vi "Untitled.vi"() -> ()   [LabVIEW 2017, in "Examples.lvlib"]
uses:
  Examples.lvlib
panel:
  in  "Bolts 3":bool
  in  "Bolts 2":bool
  in  "Valve 2":bool
  out "Pipe 2":bool
  in  "OK Button 2":bool
  out "Tank 2":dbl(slide) scale=0.0..10.0
  in  "Stop Button":bool
  out "Pipe":bool
  in  "Tank":bool
  in  "Bolts":bool
  out "Valve":bool
  in  "Switch":bool
  out "Boiler":bool
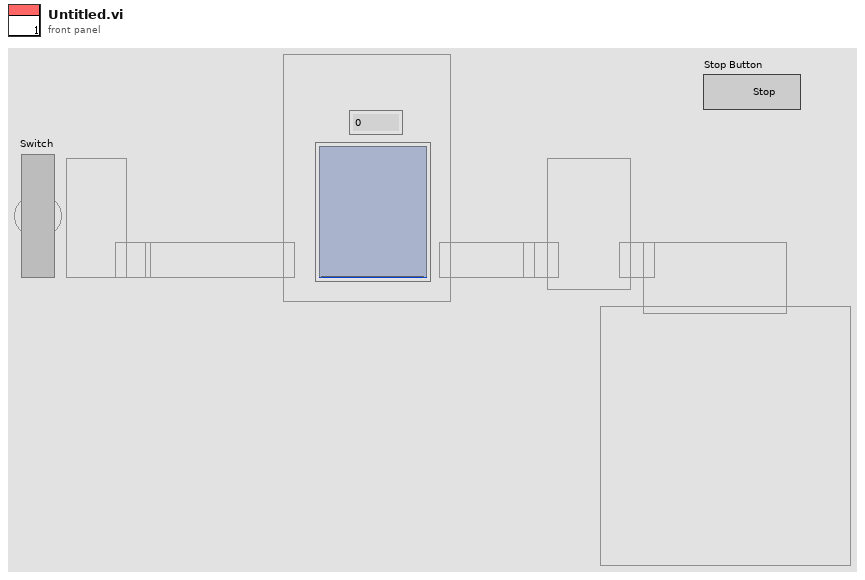
[diagram p1: front panel]
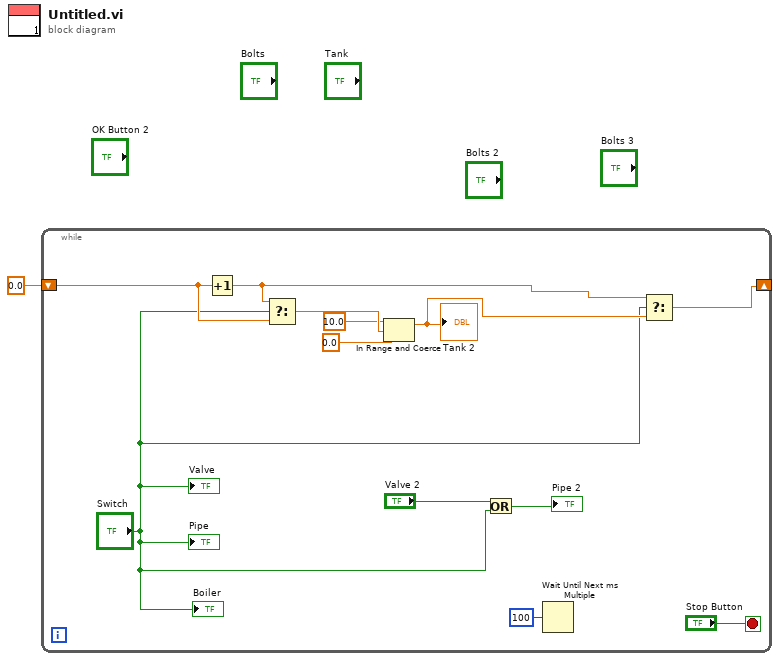
[diagram p0: block diagram]
diagram:
  n1 = while {
    shift-right: [w11] -> _
    shift-left: 0.0 -> [w12]
    stop <- "Stop Button" stop-if-true
    n2 = Increment(x=w12) -> (x+1=w9:dbl)
    n3 = Select(t=w9, s="Switch", f=w12) -> (s? t:f=w8:dbl)
    n4 = In Range and Coerce(upper limit=10.0, x=w8, lower limit=0.0) -> (coerced(x)=w5:dbl)  [unwired: 1 out]
    "Tank 2" <- w5
    n5 = Or(x="Valve 2", y="Switch") -> (x .or. y?=→"Pipe 2":bool)
    n6 = Wait Until Next ms Multiple(millisecond multiple=u32 100) -> ()  [unwired: 1 out]
    n7 = Select(t=w9, s="Switch", f=w5) -> (s? t:f=w11:dbl)
    "Valve" <- "Switch"
    "Pipe" <- "Switch"
    "Boiler" <- "Switch"
  }
